vi "Write Height.vi"(8 "error in (no error)":errorcluster, 10 "Height":dbl, 11 "Image in":refnum<class "SVGImage.lvclass">) -> (0 "error out":errorcluster, 3 "Image out":refnum<class "SVGImage.lvclass">)   [LabVIEW 2019, in "SVGImage.lvclass"]
uses:
  SVGImage.lvclass
  SVGImage.lvclass/SVGImage.ctl
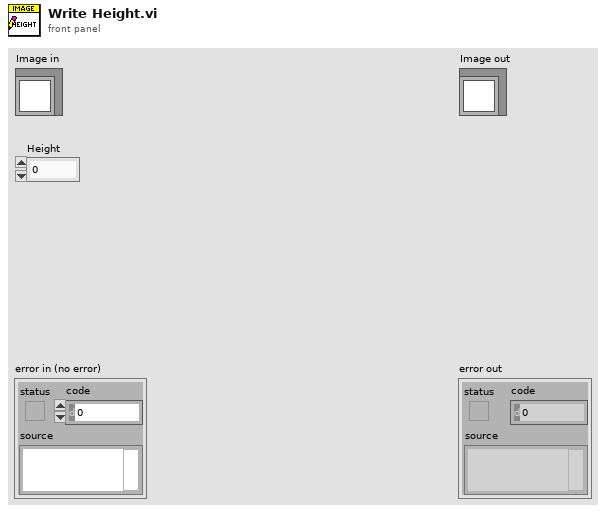
[diagram p1: front panel]
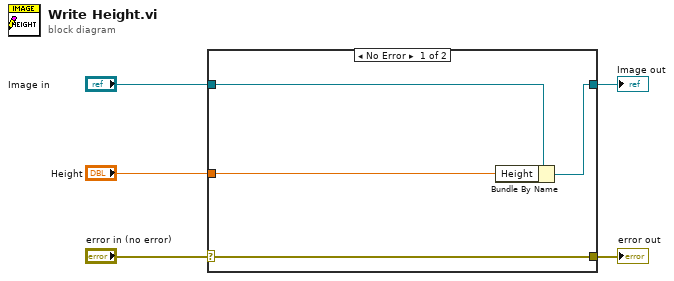
[diagram p0: block diagram]
diagram:
  n1 = case shown="No Error" "error in (no error)" {
    selector: "error in (no error)" -> [w9 w10]
    tunnel: [w9 w10] -> w4
    tunnel: [w7 w11] -> w2
    tunnel: "Image in" -> [w8 w11]
    tunnel: "Height" -> [w6 _]
    frame No Error {
      n2 = Bundle By Name(cluster=w8, "Height"=w6) -> (w7:refnum<class "SVGImage.lvclass">)
    }
    frame Error {
    }
  }
  "error out" <- w4
  "Image out" <- w2
